vi "LIA PLL to External Clock and Drive PXI_CLK10_IN.vi"() -> ()   [LabVIEW 2017]
doc: "Description:\nThis VI uses the PLL circuit to lock to an external clock, and routes it to the PXI_CLK10 signal as well. The program will continue checking for PLL lock until the user stops the program.\n\nHW Requirements:\nSystem Timing module with a PLL in the System Timing Slot of the PXI chassis\n\nConnections:\nConnect the external clock to PLL to at the CLK IN terminal."
uses:
  <instrlib>/niSync/niSync.llb/niSync Initialize (IVI).vi
panel:
  in  "Resource name":refnum<k15>="PXI1Slot2"
  in  "stop":bool
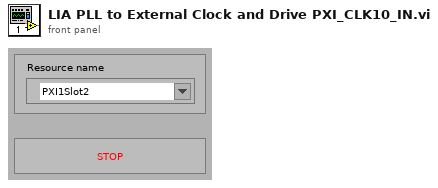
[diagram p1: front panel]
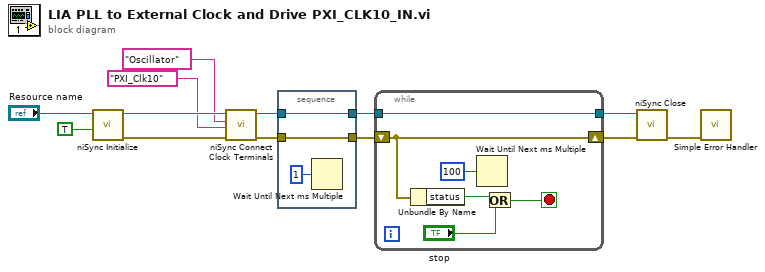
[diagram p0: block diagram]
diagram:
  n1 = call-poly <instrlib>:"niSync Initialize.vi"("reset device (F)"=TRUE ("reset device (False)"), "resource name"="Resource name") -> ("error out"=w10:errorcluster, "instrument handle out"=w11:refnum<k15>)  [unwired: 8 in]
  n2 = call <instrlib>:"niSync Connect Clock Terminals.vi"("error in (no error)"=w10, "destination terminal"="PXI_Clk10", "source terminal"="Oscillator", "instrument handle"=w11) -> ("error out"=w2:errorcluster, "instrument handle out"=w5:refnum<k15>)  [unwired: 6 in]
  n3 = stacked-sequence {
    tunnel: [w16] -> w4
    tunnel: w5 -> [w16]
    tunnel: w2 -> [w15]
    tunnel: [w15] -> w3
    frame #0 {
      n4 = Wait Until Next ms Multiple(millisecond multiple=u32 1) -> ()  [unwired: 1 out]
    }
  }
  n5 = while {
    tunnel: [w21] -> w8
    tunnel: w4 -> [w21]
    shift-right: [w18] -> w9
    shift-left: w3 -> [w18]
    stop <- w17 stop-if-true
    n6 = Unbundle By Name(w18) -> ("status"=w20:bool)
    n7 = Wait Until Next ms Multiple(millisecond multiple=u32 100) -> ()  [unwired: 1 out]
    n8 = Or(x=w20, y="stop") -> (x .or. y?=w17:bool)
  }
  n9 = call <instrlib>:"niSync Close.vi"("error in (no error)"=w9, "instrument handle"=w8) -> ("error out"=w13:errorcluster)  [unwired: 9 in]
  n10 = call <vilib>:"Simple Error Handler.vi"("error in (no error)"=w13) -> ()  [unwired: 4 in, 5 out]
